vi "lawofsineb.vi"(9 "Angle B":dbl format="%#_13g", 10 "Angle A":dbl format="%#_13g", 11 "a":dbl format="%#_13g") -> (3 "b":dbl format="%#_13g")   [LabVIEW 2018]
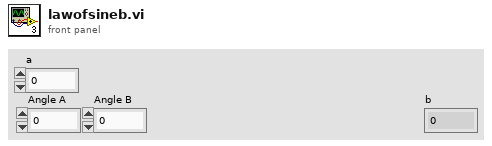
[diagram p1: front panel]
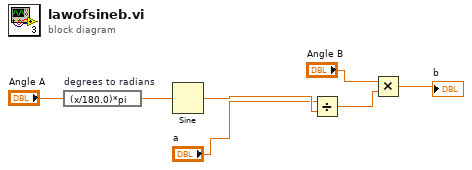
[diagram p0: block diagram]
diagram:
  n1 = expression code="(x/180.0)*pi" "degrees to radians"("Angle A") -> (w4:dbl)
  n2 = Sine(x=w4) -> (sin(x)=w2:dbl)
  n3 = Divide(x="a", y=w2) -> (x/y=w6:dbl)
  n4 = Multiply(x="Angle B", y=w6) -> (x*y=→"b":dbl)
